vi "Lidar Code XY.vi"() -> ()   [LabVIEW 2016]
uses:
  <instrlib>/Hokuyo URG Series/Public/Initialize-cRIO-USB.vi
  <instrlib>/Hokuyo URG Series/Hokuyo URG Series.lvlib
panel:
  out "XY Graph":cluster{"Y":dbl[], "Y":dbl[]}[](graph)
  in  "polar attributes (hidden)":T1={"maximum"=30000.0, "minimum"=0.0, "clip to min"=FALSE, "log?(F)"=TRUE, "grid color"=6710886, "plot color"=65280, "fmt and prec"={"format"=enum."Decimal", "precision"=0}, "visible section"=8} {"minimum" format="%0.2f"; "maximum" format="%0.2f"}
  in  "Protocol":u32(ring)=2 items=["Convert to Latest", "SCIP 1.1", "SCIP 2.0"]
  in  "ID Query?":bool=TRUE
  in  "Checksum":bool
  in  "Stop":bool
  out "Data Aquired":picture
  in  "Grid Color":u32(colorbox)=16777222
  in  "Plot Color":u32(colorbox)=6618880
  in  "Max (m)":dbl=4.1
  in  "End Point":dbl=120.0
  in  "Start Point":dbl=-120.0
  in  "Cluster Count":dbl=1.0
  in  "Encoding Width":u16(ring)=3 items=["2 Byte"=2, "3 Byte"=3]
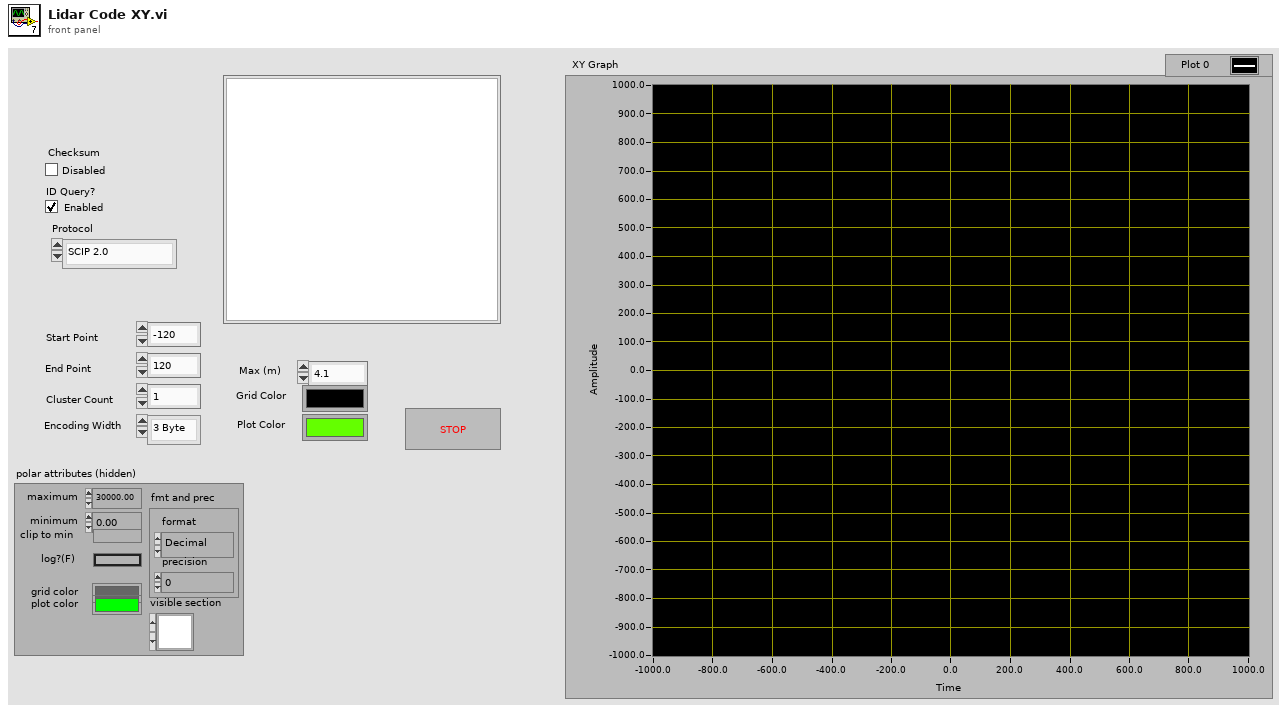
[diagram p1: front panel]
types:
  T1 = cluster{"maximum":dbl, "minimum":dbl, "clip to min":bool, "log?(F)":bool, "grid color":u32, "plot color":u32, "fmt and prec":cluster{"format":enum8{"Decimal", "Scientific", "Engineering", "Binary", "Octal", "Hex"}, "precision":u8}, "visible section":u16}
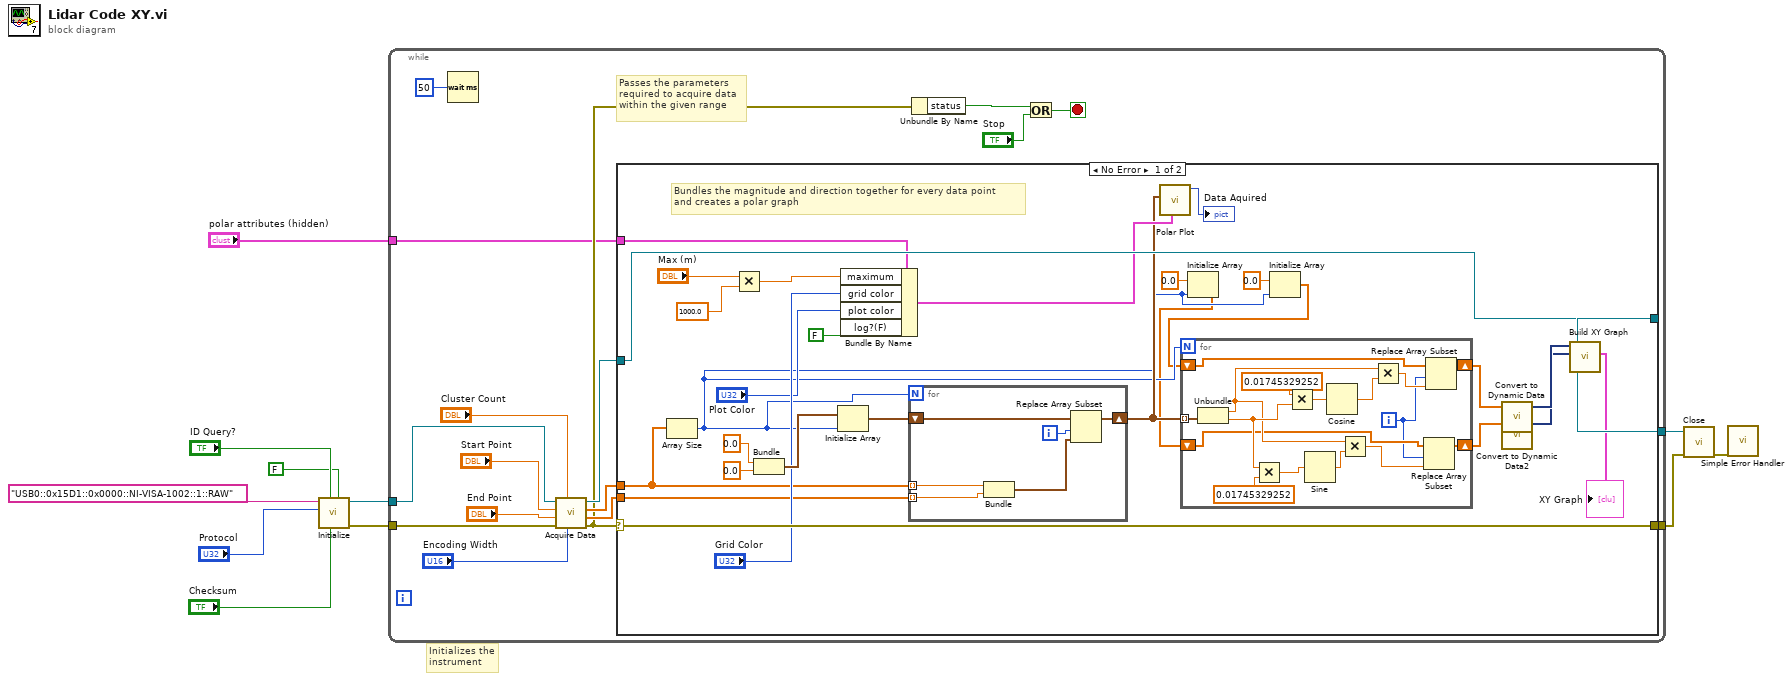
[diagram p0: block diagram]
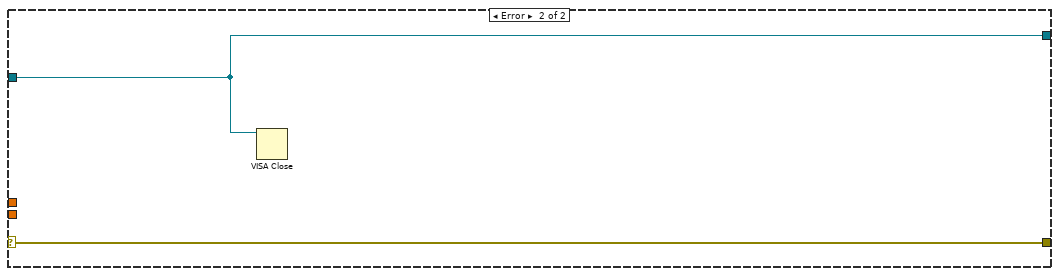
[diagram p2: hidden frame]
diagram:
  # "Initializes the instrument"
  n1 = call-poly <instrlib>:"Initialize.vi"("Reset? (F: No)"=FALSE ("Reset Instrument (Disabled)"), "Checksum (Disabled)"="Checksum", "ID Query? (Enabled)"="ID Query?", "Protocol (2: SCIP 2.0)"="Protocol", "VISA resource name"="USB0::0x15D1::0x0000::NI-VISA-1002::1::RAW") -> ("error out"=w4:errorcluster, "VISA resource name out"=w5:refnum<visa-resource-name>)  [unwired: 5 in]
  n2 = while {
    tunnel: w5 -> [w18]
    tunnel: [w13] -> w11
    tunnel: w4 -> [w17]
    tunnel: "polar attributes (hidden)" -> [w16]
    tunnel: [w12] -> w1
    stop <- w26 stop-if-true
    # "Passes the parameters\nrequired to acquire data\nwithin the given range"
    n3 = Wait (ms)(milliseconds to wait=u32 50) -> ()  [unwired: 1 out]
    n4 = call <instrlib>:"Acquire Data.vi"("Data Encoding Width (3 Byte)"="Encoding Width", "Cluster Count (1)"="Cluster Count", "error in (no error)"=w17, "End Point (120°)"="End Point", "Start Point (-120°)"="Start Point", "VISA resource name"=w18) -> ("error out"=w22:errorcluster, "Direction"=w23:dbl[], "Magnitude"=w24:dbl[], "VISA resource name out"=w25:refnum<visa-resource-name>)  [unwired: 2 in]
    n5 = case shown="No Error" w22 {
      selector: w22 -> [w54 w80]
      tunnel: [w54 w80] -> w13
      tunnel: w25 -> [w55 w79]
      tunnel: [w55 w79] -> w12
      tunnel: w24 -> [w40 _]
      tunnel: w23 -> [w41 _]
      tunnel: w16 -> [w48 _]
      frame No Error {
        # "Bundles the magnitude and direction together for every data point\nand creates a polar graph"
        n6 = Array Size(array=w40) -> (size(s)=w36:i32)
        n7 = Multiply(x="Max (m)", y=1000.0) -> (x*y=w44:dbl)
        n8 = Bundle(0.0, 0.0) -> (w51:cluster{dbl, dbl})  [unwired: 1 in]
        n9 = Initialize Array(w51, w36) -> (w50:cluster{dbl, dbl}[])
        n10 = Bundle By Name(cluster=w48, "maximum"=w44, "grid color"="Grid Color", "plot color"="Plot Color", "log?(F)"=FALSE) -> (w49:T1)
        n11 = for {
          N: w36 -> [_]
          shift-right: [w74] -> w39
          shift-left: w50 -> [w75]
          tunnel: w40 -> [w78] mode=indexing
          tunnel: w41 -> [w77] mode=indexing
          i -> [w76]
          n12 = Bundle(w78, w77) -> (w73:cluster{dbl, dbl})  [unwired: 1 in]
          n13 = Replace Array Subset(array=w75, new element=w73, index=w76) -> (w74:cluster{dbl, dbl}[])
        }
        n14 = call <vilib>:"Polar Plot.vi"("polar attributes"=w49, "data array [mag, phase (deg)]"=w39) -> ("new picture"=→"Data Aquired":picture)  [unwired: 9 in]
        n15 = Initialize Array(0.0 ("element"), w36) -> (w34:dbl[])
        n16 = Initialize Array(0.0 ("element"), w36) -> (w35:dbl[])
        n17 = for {
          N: w36 -> [_]
          tunnel: w39 -> [w72] mode=indexing
          shift-right: [w58] -> w32
          shift-left: w35 -> [w67]
          shift-right: [w57] -> w30
          shift-left: w34 -> [w60]
          i -> [w59]
          n18 = Unbundle(w72) -> (w62:dbl, w63:dbl)
          n19 = Multiply(x=w63, y=0.01745329252 ("x")) -> (x*y=w65:dbl)
          n20 = Multiply(x=0.01745329252, y=w63) -> (x*y=w69:dbl)
          n21 = Sine(x=w65) -> (sin(x)=w66:dbl)
          n22 = Cosine(x=w69) -> (cos(x)=w70:dbl)
          n23 = Multiply(x=w62, y=w66) -> (x*y=w61:dbl)
          n24 = Multiply(x=w62, y=w70) -> (x*y=w71:dbl)
          n25 = Replace Array Subset(array=w60, new element=w61, index=w59) -> (w57:dbl[])
          n26 = Replace Array Subset(array=w67, new element=w71, index=w59) -> (w58:dbl[])
        }
        n27 = call "Convert to Dynamic Data"("Array"=w32) -> ("Dynamic Data Type"=w31:dynamicdata)  [unwired: 3 in]
        n28 = call "Convert to Dynamic Data2"("Array"=w30) -> ("Dynamic Data Type"=w29:dynamicdata)  [unwired: 3 in]
        n29 = call "Build XY Graph"("Y Input"=w29, "X Input"=w31) -> ("XY Graph"=→"XY Graph":cluster{"X":dbl[], "Y":dbl[]}[])  [unwired: 8 in, 1 out]
      }
      frame Error {
        n30 = VISA Close(VISA resource name=w79) -> ()  [unwired: 1 in, 1 out]
      }
    }
    n31 = Unbundle By Name(w22) -> ("status"=w28:bool)
    n32 = Or(x=w28, y="Stop") -> (x .or. y?=w26:bool)
  }
  n33 = call <instrlib>:"Close.vi"("error in (no error)"=w11, "VISA resource name"=w1) -> ("error out"=w9:errorcluster)  [unwired: 9 in]
  n34 = call <vilib>:"Simple Error Handler.vi"("error in (no error)"=w9) -> ()  [unwired: 4 in, 5 out]
